vi "Begin.vi"(11 "Image Size":T1=enum."160x120") -> (0 "error out":errorcluster)   [LabVIEW 2012]
doc: "Called before other user functions, this VI is expected to open initial I/O refnums, load in file data, and do all program initialization. Notice that the <B>error out</B> terminal is simply used for data flow. Wiring it to other structures or subVIs ensures that this VI runs first."
uses:
  <vilib>/Rock Robotics/WPI/Camera/WPI_CameraImageSize.ctl
  <vilib>/Rock Robotics/WPI/Camera/WPI_CameraWhite Balance Values.ctl
  <vilib>/Rock Robotics/WPI/Camera/WPI_CameraExposure Values.ctl
  <vilib>/Rock Robotics/WPI/Camera/WPI_CameraFrameRate.ctl
  <vilib>/Rock Robotics/WPI/DriverStation/WPI_DriverStationRobotMode2.ctl
  <vilib>/Rock Robotics/WPI/Joystick/WPI_JoystickDeviceEnum.ctl
  <vilib>/Rock Robotics/WPI/CAN/Jaguar/SubVIs/WPI_CANJaguar_ControlMode.ctl
  <vilib>/Rock Robotics/SystemInterfaces/DIO/FPGA_DIOChannel.ctl
  Robot Global Data.vi
  <vilib>/Rock Robotics/WPI/MotorControl/WPI_MotorControlOpenCANJaguar.vi
  <vilib>/Rock Robotics/WPI/RobotDrive/WPI_RobotDriveOpen2MotorWithExistingMotors.vi
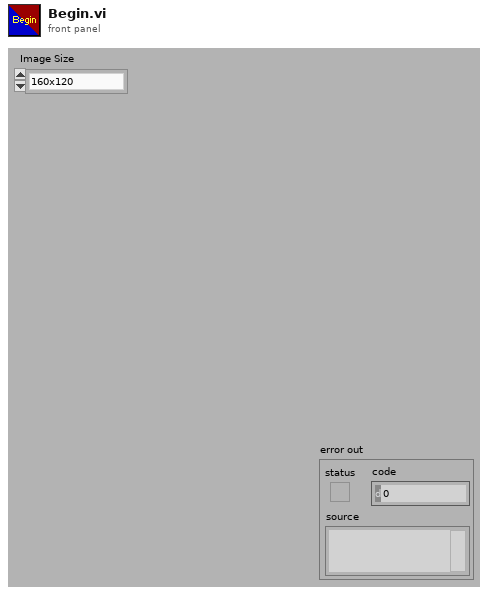
[diagram p1: front panel]
types:
  T1 = typedef "WPI_CameraImageSize.ctl" = enum16{"640x480", "320x240", "160x120"}
  T2 = typedef "FPGA_DIOChannel.ctl" = enum8{"DIO 1", "DIO 2", "DIO 3", "DIO 4", "DIO 5", "DIO 6", "DIO 7", "DIO 8", "DIO 9", "DIO 10", "DIO 11", "DIO 12", "DIO 13", "DIO 14", "Invalid"}
  T3 = typedef "WPI_CANJaguar_ControlMode.ctl" = enum8{"Percent VBus", "Current", "Speed", "Position", "Voltage"}
  T4 = typedef "WPI_JoystickDeviceEnum.ctl" = enum16{"USB 1", "USB 2", "USB 3", "USB 4", "Kinect 1", "Kinect 2"}
  T5 = typedef "WPI_DriverStationRobotMode2.ctl" = enum16{"Autonomous Disabled", "Autonomous Enabled", "Teleop Disabled", "Teleop Enabled", "Timeout", "Finish", "Test Disabled", "Test Enabled"}
  T6 = typedef "WPI_CameraFrameRate.ctl" = u32
  T7 = typedef "WPI_CameraExposure Values.ctl" = enum16{"Auto", "Flicker-free 50 Hz", "Flicker-free 60 Hz", "Hold current"}
  T8 = typedef "WPI_CameraWhite Balance Values.ctl" = enum16{"Auto", "Fixed indoor", "Fixed outdoor 1", "Fixed outdoor 2", "Fixed fluorescent 1", "Fixed fluorescent 2", "Hold current"}
  T9 = typedef "WPI_MotorControlDeviceRef.ctl" = cluster{"DeviceStatus":errorcluster, "Type":enum16{"PWM", "CAN"}, "PWM":cluster{"Digital Module":T10, "PWM Channel":T11, "DeadBand":T12}, "CAN":cluster{"Device Number":u8, "Control Mode":T3, "Semaphore":T13, "Max Vout":dbl}, "Invert":bool, "TransformRef":T14, "InvTransformRef":T14}
  T10 = typedef "FPGA_TypedefDigitalModule.ctl" = enum16{"Digital Module 1", "Digital Module 2"}
  T11 = typedef "FPGA_DIOPWMChannel.ctl" = enum8{"PWM 1", "PWM 2", "PWM 3", "PWM 4", "PWM 5", "PWM 6", "PWM 7", "PWM 8", "PWM 9", "PWM 10", "Invalid"}
  T12 = typedef "WPI_PWMDeadband.ctl" = cluster{"Name":string, "maxPositivePwm":i32, "minPositivePwm":i32, "centerPwm":i32, "maxNegativePwm":i32, "minNegativePwm":i32, "angularRange":u16}
  T13 = typedef "Semaphore RefNum" = refnum<k1>
  T14 = typedef "WPI_PWMTransform_ConPane.ctl" = refnum<vi>
  T15 = typedef "WPI_DigitalInputDevRef.ctl" = cluster{"DevStatus":errorcluster, "DIO Channel":T2, "Digital Module":T10}
  T16 = typedef "WPI_JoystickDevRef.ctl" = cluster{"Device":T4}
  T17 = typedef "WPI_CameraDevRef.ctl" = cluster{"Camera Address":string, "CameraStatus":errorcluster, "Acquire Image Notifier":refnum<notifier>}
  T18 = typedef "WPI_RobotDriveDevRef.ctl" = cluster{"DevStatus":errorcluster, "Motors[]":T9[], "Square Inputs":bool, "Max Output":dbl, "Isochronous":bool}
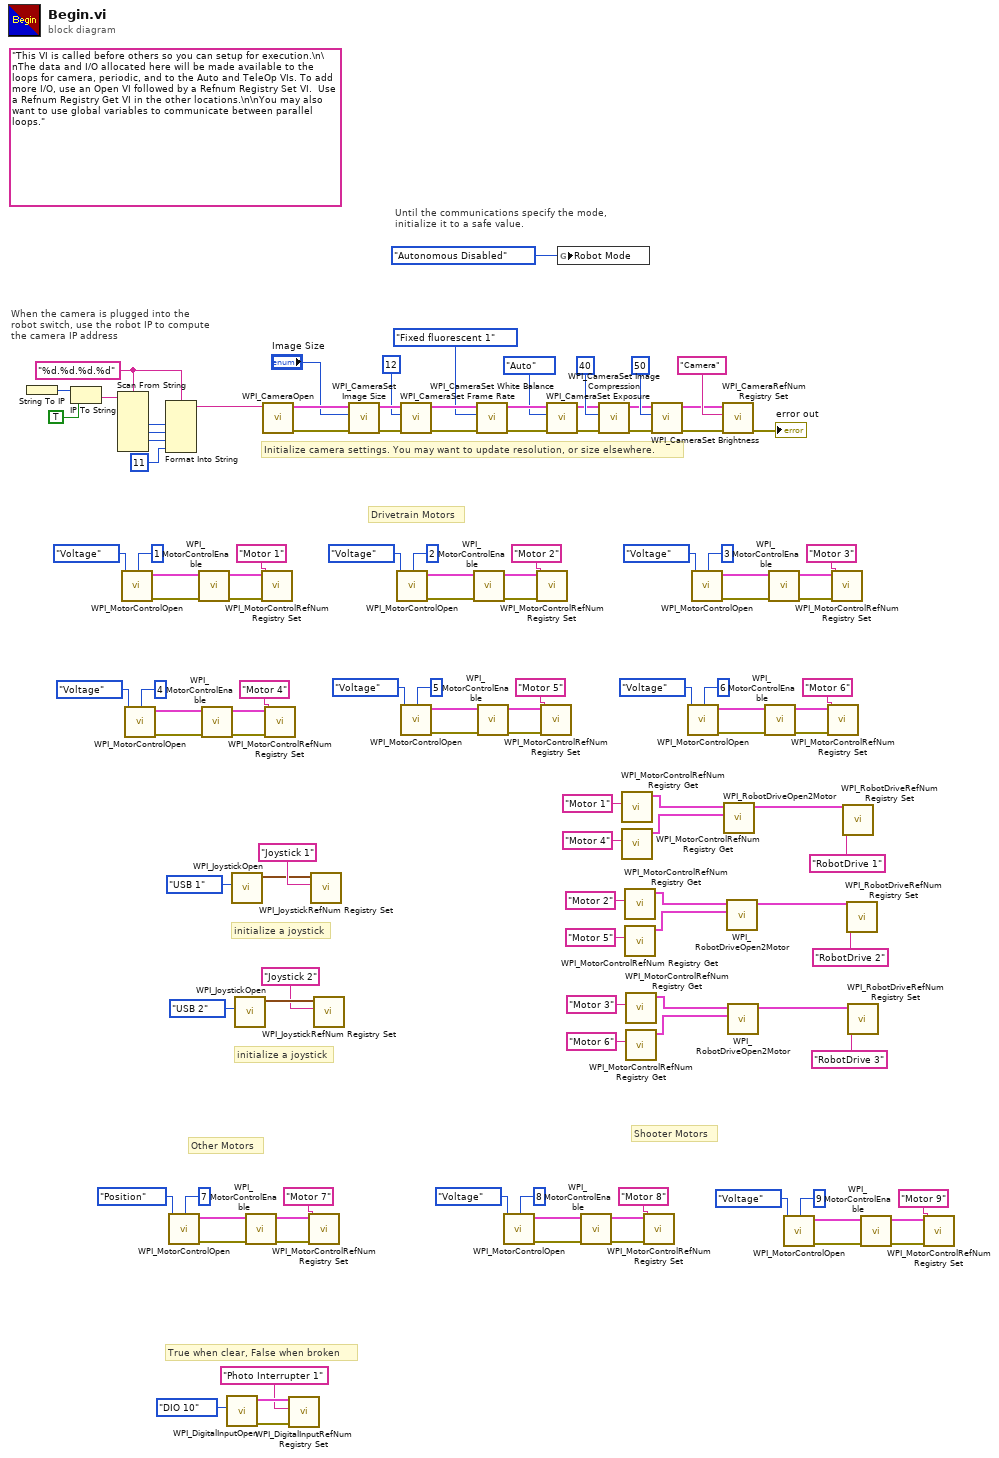
[diagram p0: block diagram]
diagram:
  w95 = "%d.%d.%d.%d" ("format string")
  (unwired) "This VI is called before others so you can setup for execution.\n\nThe data and I/O allocated here will be made available to the loops for camera, periodic, and to the Auto and TeleOp VIs. To add more I/O, use an Open VI followed by a Refnum Registry Set VI.  Use a Refnum Registry Get VI in the other locations.\n\nYou may also want to use global variables to communicate between parallel loops."
  # "True when clear, False when broken"
  # "Drivetrain Motors"
  # "Other Motors"
  # "Shooter Motors"
  # "initialize a joystick"
  # "initialize a joystick"
  # "Until the communications specify the mode,\ninitialize it to a safe value."
  # "When the camera is plugged into the\nrobot switch, use the robot IP to compute\nthe camera IP address"
  # "Initialize camera settings. You may want to update resolution, or size elsewhere."
  n1 = String To IP() -> (0:w102:u32)  [unwired: 1 in]
  n2 = IP To String(1:TRUE ("dot notation? (F)"), 2:w102) -> (0:w100:string)
  n3 = Scan From String(format string=w95, input string=w100) -> (output 1=w99:i32, output 2=w98:i32, output 3=w97:i32)  [unwired: 7 in, 3 out]
  n4 = call-poly <vilib>:"WPI_MotorControlOpen.vi"("Device Number"=u8 1, "Control Mode"=WPI_CANJaguar_ControlMode."Voltage") -> ("error out"=w88:errorcluster, "MotorControlDeviceRef"=w89:T9)  [unwired: 8 in]
  n5 = call-poly <vilib>:"WPI_MotorControlOpen.vi"("Device Number"=u8 4, "Control Mode"=WPI_CANJaguar_ControlMode."Voltage") -> ("error out"=w78:errorcluster, "MotorControlDeviceRef"=w79:T9)  [unwired: 8 in]
  n6 = Format Into String(format string=w95, w99, w98, w97, 11 ("Compression")) -> (resulting string=w93:string)  [unwired: 2 in, 1 out]
  n7 = call-poly <vilib>:"WPI_MotorControlOpen.vi"("Device Number"=u8 7, "Control Mode"=WPI_CANJaguar_ControlMode."Position") -> ("error out"=w22:errorcluster, "MotorControlDeviceRef"=w23:T9)  [unwired: 8 in]
  n8 = call <vilib>:"WPI_MotorControlEnable.vi"("error in (no error)"=w88, "CAN Jaguar Ref"=w89) -> ("error out"=w85:errorcluster, "CAN Jaguar Ref Out"=w87:T9)  [unwired: 8 in]
  n9 = call <vilib>:"WPI_MotorControlEnable.vi"("error in (no error)"=w78, "CAN Jaguar Ref"=w79) -> ("error out"=w75:errorcluster, "CAN Jaguar Ref Out"=w77:T9)  [unwired: 8 in]
  n10 = call <vilib>:"WPI_DigitalInputOpen.vi"("DIO Channel"=FPGA_DIOChannel."DIO 10") -> ("error out"=w1:errorcluster, "DigitalInputDevRef"=w3:T15)  [unwired: 9 in]
  n11 = call <vilib>:"WPI_JoystickOpen.vi"("JoystickDevice"=WPI_JoystickDeviceEnum."USB 1") -> ("JoystickDevRef"=w83:T16)  [unwired: 10 in]
  n12 = call <vilib>:"WPI_JoystickOpen.vi"("JoystickDevice"=WPI_JoystickDeviceEnum."USB 2") -> ("JoystickDevRef"=w45:T16)  [unwired: 10 in]
  n13 = call <vilib>:"WPI_MotorControlEnable.vi"("error in (no error)"=w22, "CAN Jaguar Ref"=w23) -> ("error out"=w19:errorcluster, "CAN Jaguar Ref Out"=w21:T9)  [unwired: 8 in]
  n14 = call <vilib>:"WPI_MotorControlRefNum Registry Set.vi"("error in (no error)"=w85, "refnum name"="Motor 1", "MotorControlDevRef"=w87) -> ()  [unwired: 7 in, 2 out]
  n15 = call <vilib>:"WPI_CameraOpen.vi"("Camera Address"=w93) -> ("error out"=w114:errorcluster, "CameraDevRef"=w115:T17)  [unwired: 1 in, 8 out]
  n16 = call <vilib>:"WPI_MotorControlRefNum Registry Set.vi"("error in (no error)"=w75, "refnum name"="Motor 4", "MotorControlDevRef"=w77) -> ()  [unwired: 7 in, 2 out]
  n17 = call <vilib>:"WPI_DigitalInputRefNum Registry Set.vi"("error in (no error)"=w1, "refnum name"="Photo Interrupter 1", "DigitalInputDevRef"=w3) -> ()  [unwired: 7 in, 2 out]
  n18 = call <vilib>:"WPI_MotorControlRefNum Registry Set.vi"("error in (no error)"=w19, "refnum name"="Motor 7", "MotorControlDevRef"=w21) -> ()  [unwired: 7 in, 2 out]
  n19 = call <vilib>:"WPI_JoystickRefNum Registry Set.vi"("refnum name"="Joystick 1", "JoystickDevRef"=w83) -> ()  [unwired: 8 in, 2 out]
  n20 = call <vilib>:"WPI_JoystickRefNum Registry Set.vi"("refnum name"="Joystick 2", "JoystickDevRef"=w45) -> ()  [unwired: 8 in, 2 out]
  n21 = call <vilib>:"WPI_CameraSet Image Size.vi"("error in (no error)"=w114, "Image Size"="Image Size", "CameraDevRef"=w115) -> ("error out"=w113:errorcluster, "CameraDevRef Out"=w116:T17)  [unwired: 7 out]
  n22 = call-poly <vilib>:"WPI_MotorControlOpen.vi"("Device Number"=u8 2, "Control Mode"=WPI_CANJaguar_ControlMode."Voltage") -> ("error out"=w71:errorcluster, "MotorControlDeviceRef"=w72:T9)  [unwired: 8 in]
  n23 = call <vilib>:"WPI_CameraSet Frame Rate.vi"("error in (no error)"=w113, "Frame Rate (fps)"=T6 12, "CameraDevRef"=w116) -> ("error out"=w112:errorcluster, "CameraDevRef Out"=w118:T17)  [unwired: 7 out]
  n24 = call-poly <vilib>:"WPI_MotorControlOpen.vi"("Device Number"=u8 5, "Control Mode"=WPI_CANJaguar_ControlMode."Voltage") -> ("error out"=w64:errorcluster, "MotorControlDeviceRef"=w65:T9)  [unwired: 8 in]
  n25 = call <vilib>:"WPI_MotorControlEnable.vi"("error in (no error)"=w71, "CAN Jaguar Ref"=w72) -> ("error out"=w68:errorcluster, "CAN Jaguar Ref Out"=w70:T9)  [unwired: 8 in]
  n26 = call <vilib>:"WPI_CameraSet White Balance.vi"("error in (no error)"=w112, "White Balance"=WPI_CameraWhite_Balance_Values."Fixed fluorescent 1", "CameraDevRef"=w118) -> ("error out"=w111:errorcluster, "CameraDevRef Out"=w117:T17)  [unwired: 7 out]
  n27 = call <vilib>:"WPI_MotorControlEnable.vi"("error in (no error)"=w64, "CAN Jaguar Ref"=w65) -> ("error out"=w61:errorcluster, "CAN Jaguar Ref Out"=w63:T9)  [unwired: 8 in]
  n28 = call-poly <vilib>:"WPI_MotorControlOpen.vi"("Device Number"=u8 8, "Control Mode"=WPI_CANJaguar_ControlMode."Voltage") -> ("error out"=w15:errorcluster, "MotorControlDeviceRef"=w16:T9)  [unwired: 8 in]
  n29 = call <vilib>:"WPI_MotorControlRefNum Registry Set.vi"("error in (no error)"=w68, "refnum name"="Motor 2", "MotorControlDevRef"=w70) -> ()  [unwired: 7 in, 2 out]
  n30 = call <vilib>:"WPI_MotorControlRefNum Registry Set.vi"("error in (no error)"=w61, "refnum name"="Motor 5", "MotorControlDevRef"=w63) -> ()  [unwired: 7 in, 2 out]
  n31 = call <vilib>:"WPI_CameraSet Exposure.vi"("error in (no error)"=w111, "Exposure"=WPI_CameraExposure_Values."Auto", "CameraDevRef"=w117) -> ("error out"=w110:errorcluster, "CameraDevRef Out"=w120:T17)  [unwired: 7 out]
  n32 = global write "Robot Global Data.vi" "Robot Mode"(WPI_DriverStationRobotMode2."Autonomous Disabled" ("Robot Mode")) -> ()
  n33 = call <vilib>:"WPI_MotorControlEnable.vi"("error in (no error)"=w15, "CAN Jaguar Ref"=w16) -> ("error out"=w12:errorcluster, "CAN Jaguar Ref Out"=w14:T9)  [unwired: 8 in]
  n34 = call <vilib>:"WPI_CameraSet Image Compression.vi"("error in (no error)"=w110, "Compression"=40, "CameraDevRef"=w120) -> ("error out"=w109:errorcluster, "CameraDevRef Out"=w119:T17)  [unwired: 7 out]
  n35 = call <vilib>:"WPI_MotorControlRefNum Registry Get.vi"("refnum name"="Motor 1") -> ("MotorControlDevRef"=w43:T9)  [unwired: 9 in, 1 out]
  n36 = call <vilib>:"WPI_MotorControlRefNum Registry Get.vi"("refnum name"="Motor 4") -> ("MotorControlDevRef"=w42:T9)  [unwired: 9 in, 1 out]
  n37 = call <vilib>:"WPI_MotorControlRefNum Registry Get.vi"("refnum name"="Motor 2") -> ("MotorControlDevRef"=w39:T9)  [unwired: 9 in, 1 out]
  n38 = call <vilib>:"WPI_MotorControlRefNum Registry Get.vi"("refnum name"="Motor 5") -> ("MotorControlDevRef"=w38:T9)  [unwired: 9 in, 1 out]
  n39 = call <vilib>:"WPI_MotorControlRefNum Registry Get.vi"("refnum name"="Motor 3") -> ("MotorControlDevRef"=w35:T9)  [unwired: 9 in, 1 out]
  n40 = call <vilib>:"WPI_MotorControlRefNum Registry Get.vi"("refnum name"="Motor 6") -> ("MotorControlDevRef"=w34:T9)  [unwired: 9 in, 1 out]
  n41 = call <vilib>:"WPI_MotorControlRefNum Registry Set.vi"("error in (no error)"=w12, "refnum name"="Motor 8", "MotorControlDevRef"=w14) -> ()  [unwired: 7 in, 2 out]
  n42 = call <vilib>:"WPI_CameraSet Brightness.vi"("error in (no error)"=w109, "Brightness"=50, "CameraDevRef"=w119) -> ("error out"=w107:errorcluster, "CameraDevRef Out"=w108:T17)  [unwired: 7 out]
  n43 = call-poly <vilib>:"WPI_MotorControlOpen.vi"("Device Number"=u8 6, "Control Mode"=WPI_CANJaguar_ControlMode."Voltage") -> ("error out"=w50:errorcluster, "MotorControlDeviceRef"=w51:T9)  [unwired: 8 in]
  n44 = call-poly <vilib>:"WPI_MotorControlOpen.vi"("Device Number"=u8 3, "Control Mode"=WPI_CANJaguar_ControlMode."Voltage") -> ("error out"=w57:errorcluster, "MotorControlDeviceRef"=w58:T9)  [unwired: 8 in]
  n45 = call <vilib>:"WPI_CameraRefNum Registry Set.vi"("error in (no error)"=w107, "refnum name"="Camera", "CameraDevRef"=w108) -> ("error out"=→"error out":errorcluster)  [unwired: 8 out]
  n46 = call-poly <vilib>:"WPI_RobotDriveOpen2Motor.vi"("Right Motor Dev Ref"=w42, "Left Motor Dev Ref"=w43) -> ("RobotDriveDevRef"=w31:T18)  [unwired: 8 in, 1 out]
  n47 = call-poly <vilib>:"WPI_RobotDriveOpen2Motor.vi"("Right Motor Dev Ref"=w38, "Left Motor Dev Ref"=w39) -> ("RobotDriveDevRef"=w30:T18)  [unwired: 8 in, 1 out]
  n48 = call-poly <vilib>:"WPI_RobotDriveOpen2Motor.vi"("Right Motor Dev Ref"=w34, "Left Motor Dev Ref"=w35) -> ("RobotDriveDevRef"=w29:T18)  [unwired: 8 in, 1 out]
  n49 = call <vilib>:"WPI_MotorControlEnable.vi"("error in (no error)"=w50, "CAN Jaguar Ref"=w51) -> ("error out"=w47:errorcluster, "CAN Jaguar Ref Out"=w49:T9)  [unwired: 8 in]
  n50 = call <vilib>:"WPI_MotorControlEnable.vi"("error in (no error)"=w57, "CAN Jaguar Ref"=w58) -> ("error out"=w54:errorcluster, "CAN Jaguar Ref Out"=w56:T9)  [unwired: 8 in]
  n51 = call-poly <vilib>:"WPI_MotorControlOpen.vi"("Device Number"=u8 9, "Control Mode"=WPI_CANJaguar_ControlMode."Voltage") -> ("error out"=w8:errorcluster, "MotorControlDeviceRef"=w9:T9)  [unwired: 8 in]
  n52 = call <vilib>:"WPI_MotorControlRefNum Registry Set.vi"("error in (no error)"=w47, "refnum name"="Motor 6", "MotorControlDevRef"=w49) -> ()  [unwired: 7 in, 2 out]
  n53 = call <vilib>:"WPI_MotorControlRefNum Registry Set.vi"("error in (no error)"=w54, "refnum name"="Motor 3", "MotorControlDevRef"=w56) -> ()  [unwired: 7 in, 2 out]
  n54 = call <vilib>:"WPI_RobotDriveRefNum Registry Set.vi"("refnum name"="RobotDrive 1", "RobotDriveDevRef"=w31) -> ()  [unwired: 8 in, 2 out]
  n55 = call <vilib>:"WPI_RobotDriveRefNum Registry Set.vi"("refnum name"="RobotDrive 2", "RobotDriveDevRef"=w30) -> ()  [unwired: 8 in, 2 out]
  n56 = call <vilib>:"WPI_RobotDriveRefNum Registry Set.vi"("refnum name"="RobotDrive 3", "RobotDriveDevRef"=w29) -> ()  [unwired: 8 in, 2 out]
  n57 = call <vilib>:"WPI_MotorControlEnable.vi"("error in (no error)"=w8, "CAN Jaguar Ref"=w9) -> ("error out"=w5:errorcluster, "CAN Jaguar Ref Out"=w7:T9)  [unwired: 8 in]
  n58 = call <vilib>:"WPI_MotorControlRefNum Registry Set.vi"("error in (no error)"=w5, "refnum name"="Motor 9", "MotorControlDevRef"=w7) -> ()  [unwired: 7 in, 2 out]
